vi "Subpanel call-ROI entry screen.vi"(8 "error in":errorcluster, 11 "Experiment folder path":path) -> (0 "error out":errorcluster)   [LabVIEW 2017]
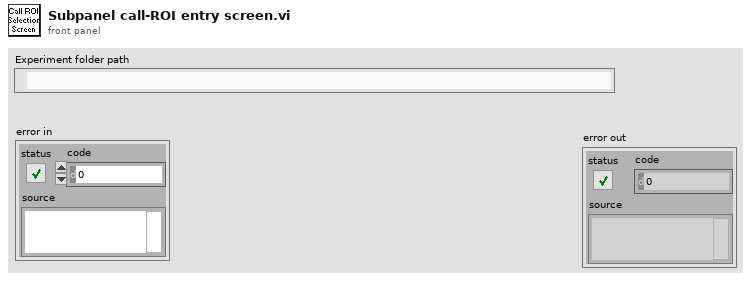
[diagram p1: front panel]
types:
  T1 = enum8{"Enabled", "Disabled", "Disabled and Grayed Out"}
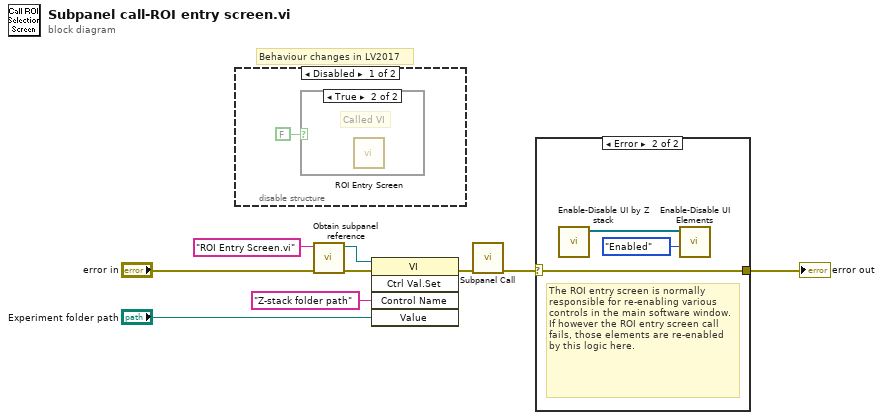
[diagram p0: block diagram]
diagram:
  # "Behaviour changes in LV2017"
  n1 = disable-structure shown="Disabled" {
    frame Disabled {
      n2 = case shown="True" FALSE {
        frame False {
        }
        frame True {
          # "Called VI"
          n3 = call "ROI Entry Screen.vi"() -> ()  [unwired: 12 in]
        }
      }
    }
    frame Enabled {
    }
  }
  n4 = call "Obtain subpanel reference.vi"("error in (no error)"="error in", "Subpanel VI name (plus \".vi\" file extension)"="ROI Entry Screen.vi" ("name or relative path")) -> ("error out"=w9:errorcluster, "Subpanel VI ref"=w8:refnum<vi>)  [unwired: 8 in]
  n5 = invoke class="VI" method="Ctrl Val.Set"(reference=w8, error in=w9, "Control Name"="Z-stack folder path", "Value"="Experiment folder path") -> (error out=w6:errorcluster)  [unwired: 1 in, 4 out]
  n6 = call "Subpanel Call.vi"("error in (no error)"=w6) -> ("error out"=w2:errorcluster)  [unwired: 10 in]
  n7 = case shown="Error" w2 {
    selector: w2 -> [w11 w12]
    tunnel: [w11 w12] -> w1
    frame No Error {
    }
    frame Error {
      # "The ROI entry screen is normally responsible for re-enabling various controls in the main software window.\nIf however the ROI entry screen call fails, those elements are re-enabled by this logic here."
      n8 = call "Enable-Disable UI by Z stack.vi"() -> ("Controls refs to enable/disable"=w14:refnum<vi>[])  [unwired: 11 in]
      n9 = call "Enable-Disable UI Elements.vi"("Enable/Disable"=T1."Enabled", "Ctrl ref's"=w14) -> ()  [unwired: 9 in, 1 out]
    }
  }
  "error out" <- w1
